vi "copy.vi"(6 "error in (no error)":errorcluster, 9 "Image in":T1) -> (0 "error out":errorcluster, 2 "copy":T1, 3 "original":T1)   [LabVIEW 2024, in "Vision.lvlib"]
uses:
  Vision.lvlib
  <vilib>/vision/Image Controls.llb/IMAQ Image.ctl
  bin/Vision.dll
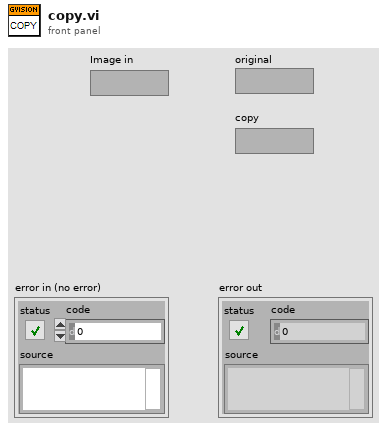
[diagram p1: front panel]
types:
  T1 = typedef "IMAQ Image.ctl" = refnum<image>
  T2 = enum32{"Map Pixel Pointer", "Unmap Pixel Pointer", "Get Pixels Infos"}
  T3 = typedef "Image Type" = u32
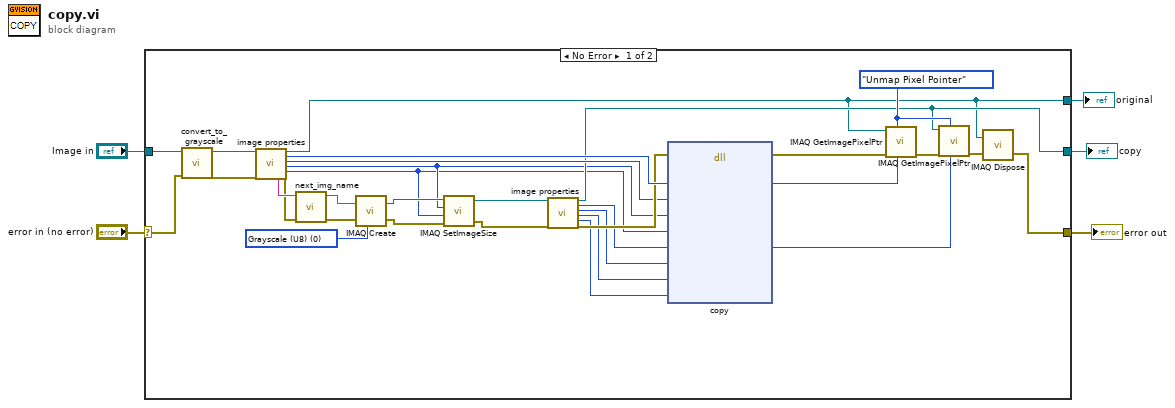
[diagram p0: block diagram]
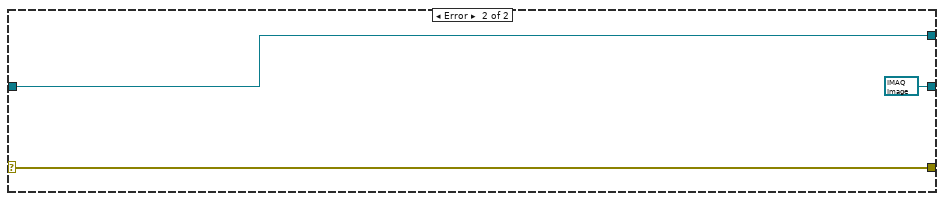
[diagram p2: hidden frame]
diagram:
  n1 = case shown="No Error" "error in (no error)" {
    selector: "error in (no error)" -> [w29 w39]
    tunnel: "Image in" -> [w30 w38]
    tunnel: [w36 w39] -> w3
    tunnel: [w13 T1 refnum ("Image out")] -> w2
    tunnel: [w6 w38] -> w1
    frame No Error {
      w31 = T2."Unmap Pixel Pointer" ("Function")
      w35 = T3 0 items=["Grayscale (U8)", "Grayscale (I16)", "Grayscale (SGL)", "Complex (CSG)", "RGB (U32)", "HSL (U32)", "RGB (U64)", "Grayscale (U16)"] ("Image Type")
      n2 = call "convert_to_grayscale.vi"("error in (no error)"=w29, "Image in"=w30) -> ("error out"=w27:errorcluster, "Image out"=w28:T1)  [unwired: 8 in]
      n3 = call "image properties.vi"("Image in"=w28, "error in (no error)"=w27) -> ("Image Name"=w12:string, "Image out"=w6:T1, "Pixel Pointer out"=w22:u64, "Line Width"=w20:i32, "X Resolution"=w8:i32, "Y Resolution"=w7:i32, "error out"=w10:errorcluster)  [unwired: 10 in, 1 out]
      n4 = call "next_img_name.vi"("error in (no error)"=w10, "name in"=w12) -> ("error out"=w9:errorcluster, "name out"=w11:string)  [unwired: 8 in]
      n5 = call "IMAQ Create"("Image Name"=w11, "Image Type"=w35, "error in (no error)"=w9) -> ("New Image"=w26:T1, "error out"=w25:errorcluster)  [unwired: 2 in]
      n6 = call "IMAQ SetImageSize"("error in (no error)"=w25, "Y Resolution"=w7, "X Resolution"=w8, "Image"=w26) -> ("error out"=w23:errorcluster, "Image Out"=w24:T1)  [unwired: 1 in]
      n7 = call "image properties.vi"("Image in"=w24, "error in (no error)"=w23) -> ("Image out"=w13:T1, "Pixel Pointer out"=w19:u64, "Line Width"=w18:i32, "X Resolution"=w17:i32, "Y Resolution"=w16:i32, "error out"=w21:errorcluster)  [unwired: 10 in, 2 out]
      n8 = dll-call lib="C:/Users/cfang/Desktop/nebraska-silicon-lab/pixel-gantry-control/Gantry/Shared Components/bin/Vision.dll" fn="copy"(error in=w21, "src_imgPtr"=w22, "src_imgLineWidth"=w20, "src_imgWidth"=w8, "src_imgHeight"=w7, "dst_imgPtr"=w19, "dst_imgLineWidth"=w18, "dst_imgWidth"=w17, "dst_imgHeight"=w16) -> (error out=w33:errorcluster, "src_imgPtr"=w15:u64, "dst_imgPtr"=w14:u64)  [unwired: 9 in, 1 out]
      n9 = call "IMAQ GetImagePixelPtr"("Pixel Pointer in"=w15, "Function"=w31, "error in (no error)"=w33, "Image"=w6) -> ("error out"=w34:errorcluster)  [unwired: 2 in, 5 out]
      n10 = call "IMAQ GetImagePixelPtr"("Pixel Pointer in"=w14, "Function"=w31, "error in (no error)"=w34, "Image"=w13) -> ("error out"=w32:errorcluster)  [unwired: 2 in, 5 out]
      n11 = call "IMAQ Dispose"("Image"=w6, "error in (no error)"=w32) -> ("error out"=w36:errorcluster)  [unwired: 4 in]
    }
    frame Error {
    }
  }
  "copy" <- w2
  "error out" <- w3
  "original" <- w1
